vi "Register_Variable_Status_Refnum.vi"(8 "error in (no error)":errorcluster, 10 "Variable Status Refnum":refnum<vi>, 11 "ExperimentVariables in":refnum<class "ExperimentVariables.lvclass">) -> (0 "error out":errorcluster, 3 "ExperimentVariables out":refnum<class "ExperimentVariables.lvclass">)   [LabVIEW 2013]
uses:
  ExperimentVariables.lvclass
  Variable_Status.ctl
  current_variables_table.ctl
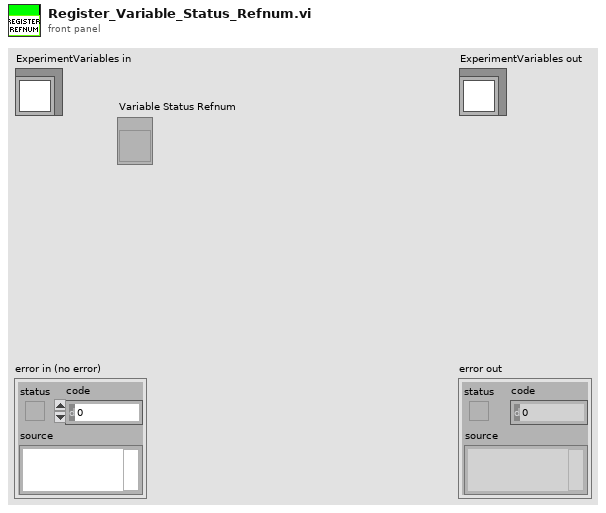
[diagram p1: front panel]
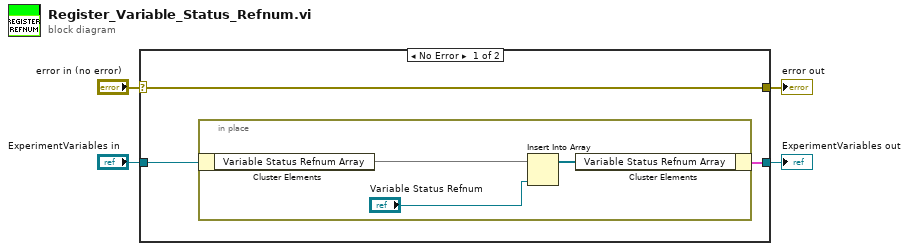
[diagram p0: block diagram]
diagram:
  n1 = case shown="No Error" "error in (no error)" {
    selector: "error in (no error)" -> [w7 w12]
    tunnel: [w7 w12] -> w3
    tunnel: [w5 w11] -> w1
    tunnel: "ExperimentVariables in" -> [w6 w11]
    frame No Error {
      n2 = in-place {
        n3 = in-place-cluster #1(w6) -> ("Variable Status Refnum Array"=w10)
        n4 = Insert Into Array(array=w10, new element="Variable Status Refnum") -> (w9:refnum<vi>[])  [unwired: 1 in]
        n5 = in-place-cluster #1("Variable Status Refnum Array"=w9) -> (w5:cluster{})
      }
    }
    frame Error {
    }
  }
  "error out" <- w3
  "ExperimentVariables out" <- w1
